vi "Write Sound Queue.vi"(8 "error in (no error)":errorcluster, 10 "Sound Queue":refnum<queue>, 11 "Electrophysiology in":refnum<class "Electrophysiology.lvclass">) -> (0 "error out":errorcluster, 3 "Electrophysiology out":refnum<class "Electrophysiology.lvclass">)   [LabVIEW 2014, in "Electrophysiology.lvclass"]
uses:
  Electrophysiology.lvclass
  Electrophysiology.lvclass/Electrophysiology.ctl
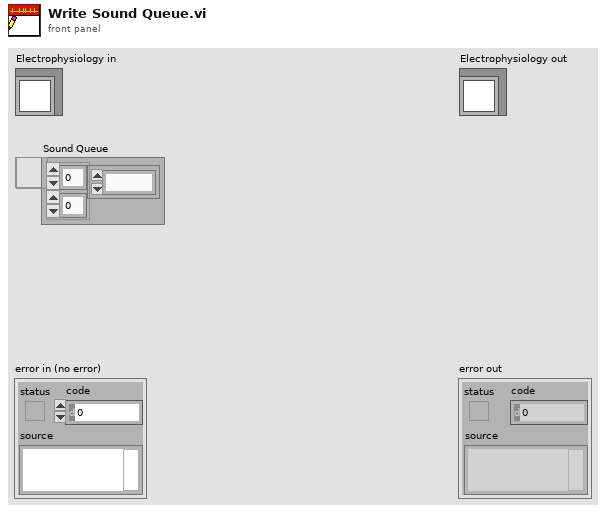
[diagram p1: front panel]
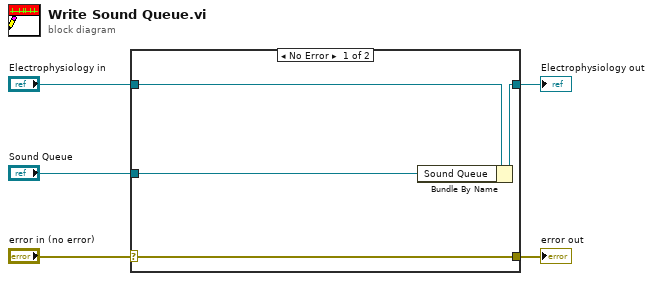
[diagram p0: block diagram]
diagram:
  n1 = case shown="No Error" "error in (no error)" {
    selector: "error in (no error)" -> [w9 w10]
    tunnel: [w9 w10] -> w4
    tunnel: [w7 w11] -> w2
    tunnel: "Electrophysiology in" -> [w8 w11]
    tunnel: "Sound Queue" -> [w6 _]
    frame No Error {
      n2 = Bundle By Name(cluster=w8, "Sound Queue"=w6) -> (w7:refnum<class "Electrophysiology.lvclass">)
    }
    frame Error {
    }
  }
  "error out" <- w4
  "Electrophysiology out" <- w2
